vi "Replace Tag.vi"(4 "Litt/BigEnd":bool, 6 "Tag":T1, 8 "Image Data in":u8[](array[numeric])) -> (3 "Image Data Out":u8[](array[numeric]))   [LabVIEW 2013, in "Tiff reader.lvlib"]
doc: "This .vi replaces a tag in the Image Data Stream."
uses:
  Tiff reader.lvlib
  IFD Entry.ctl
  FieldTypes.ctl
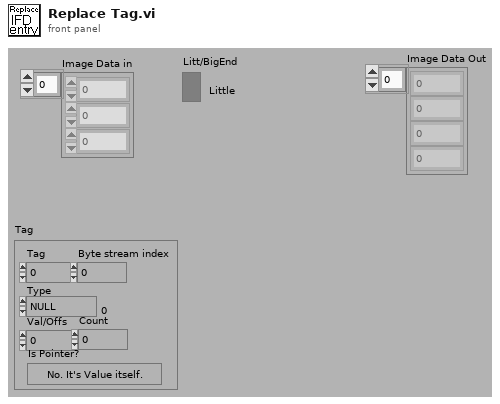
[diagram p1: front panel]
types:
  T1 = typedef "Tiff reader.lvlib/IFD Entry.ctl" = cluster{"Tag":u16, "Type":T2, "Count":u32, "Val/Offs":u32, "Is Pointer?":bool, "Byte stream index":i32}
  T2 = typedef "Tiff reader.lvlib/FieldTypes.ctl" = enum16{"NULL", "U8", "ASCII7", "U16", "U32", "RATIONAL", "SByte(I8)", "Undef(8Bit)", "I16", "I32", "SRat(4B:4B)", "SGL(4Byte)", "DBL(8Byte)"}
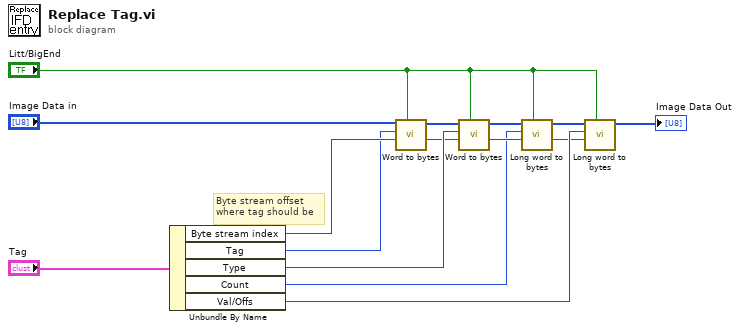
[diagram p0: block diagram]
diagram:
  # "Byte stream offset\nwhere tag should be"
  n1 = Unbundle By Name("Tag") -> ("Byte stream index"=w15:i32, "Tag"=w5:u16, "Type"=w8:T2, "Count"=w9:u32, "Val/Offs"=w14:u32)
  n2 = call "Word to bytes.vi"("Litt/BigEnd"="Litt/BigEnd", "Index"=w15, "Word"=w5, "Image Data in"="Image Data in") -> ("Index+2"=w7:i32, "Image Data out"=w6:u8[])  [unwired: 4 out]
  n3 = call "Word to bytes.vi"("Litt/BigEnd"="Litt/BigEnd", "Index"=w7, "Word"=w8, "Image Data in"=w6) -> ("Index+2"=w10:i32, "Image Data out"=w12:u8[])  [unwired: 4 out]
  n4 = call "Long word to bytes.vi"("Litt/BigEnd"="Litt/BigEnd", "Index"=w10, "U32"=w9, "Image Data in"=w12) -> ("Index+4"=w11:i32, "Image Data out"=w13:u8[])  [unwired: 4 out]
  n5 = call "Long word to bytes.vi"("Litt/BigEnd"="Litt/BigEnd", "Index"=w11, "U32"=w14, "Image Data in"=w13) -> ("Image Data out"=→"Image Data Out":u8[])  [unwired: 5 out]
